vi "Jones_Manual_Rudder.vi"(0 "Full Port":bool, 1 "Port":bool, 2 "Starboard":bool, 3 "Full Starboard":bool, 4 "Array":u8[](array[numeric])) -> (6 "Array 2":u8[](array[numeric]))   [LabVIEW 2011]
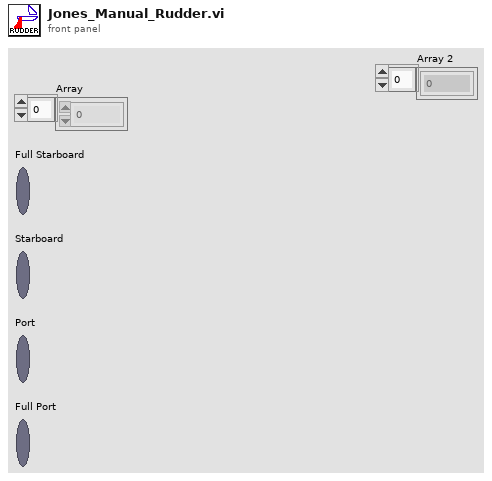
[diagram p1: front panel]
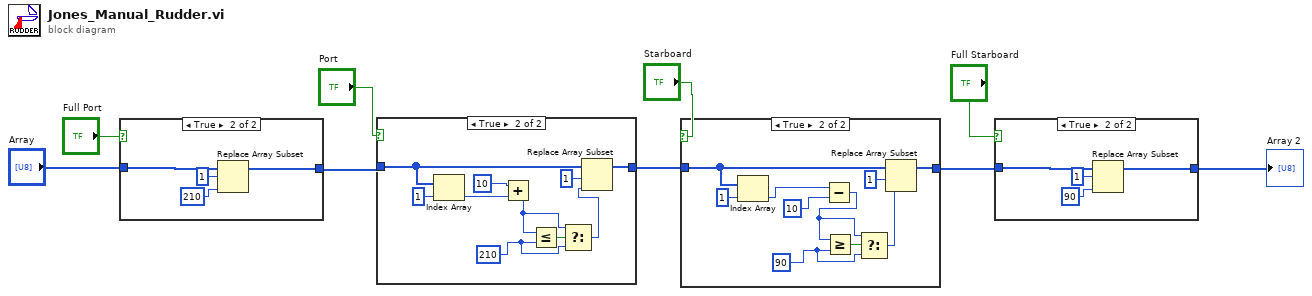
[diagram p0: block diagram]
diagram:
  n1 = case shown="True" "Full Port" {
    tunnel: "Array" -> [w10 w14]
    tunnel: [w10 w12] -> w6
    frame False {
    }
    frame True {
      n2 = Replace Array Subset(array=w14, new element=u8 210 ("new element/subarray"), index=1) -> (w12:u8[])
    }
  }
  n3 = case shown="True" "Port" {
    tunnel: w6 -> [w15 w24]
    tunnel: [w15 w25] -> w4
    frame False {
    }
    frame True {
      w16 = 210
      n4 = Index Array(array=w24, index=1) -> (element=w22:u8)
      n5 = Add(x=u8 10, y=w22) -> (x+y=w18:u8)
      n6 = Less Or Equal?(x=w18, y=w16) -> (x <= y?=w19:bool)
      n7 = Select(t=w18, s=w19, f=w16) -> (s? t:f=w17:i32)
      n8 = Replace Array Subset(array=w24, new element=w17, index=1) -> (w25:u8[])
    }
  }
  n9 = case shown="True" "Starboard" {
    tunnel: w4 -> [w26 w35]
    tunnel: [w26 w36] -> w2
    frame False {
    }
    frame True {
      w27 = 90
      n10 = Index Array(array=w35, index=1) -> (element=w31:u8)
      n11 = Subtract(x=w31, y=u8 10 ("x")) -> (x-y=w28:u8)
      n12 = Greater Or Equal?(x=w28, y=w27) -> (x >= y?=w29:bool)
      n13 = Select(t=w28, s=w29, f=w27) -> (s? t:f=w32:i32)
      n14 = Replace Array Subset(array=w35, new element=w32, index=1) -> (w36:u8[])
    }
  }
  n15 = case shown="True" "Full Starboard" {
    tunnel: w2 -> [w37 w41]
    tunnel: [w37 w39] -> w1
    frame False {
    }
    frame True {
      n16 = Replace Array Subset(array=w41, new element=u8 90 ("new element/subarray"), index=1) -> (w39:u8[])
    }
  }
  "Array 2" <- w1
